vi "ConfigureDlg.vi"(8 "error in (no error)":errorcluster, 11 "MultiBandState in":refnum<class "MultiBandState.lvclass">) -> (0 "error out":errorcluster, 2 "Changed":bool, 3 "MultiBandState out":refnum<class "MultiBandState.lvclass">)   [LabVIEW 2014, in "Functions.lvlib" / "MultiBandState.lvclass"]
uses:
  MultiBandState.lvclass
  TypeDefs/clMultiBandConfig.ctl
  TypeDefs/MultiBandConfig.ctl
  MultiBandState.lvclass/MultiBandState.ctl
  FunctionBaseClass/FunctionBase.lvclass/FunctionBase.ctl
  FunctionBaseClass/Accessors/Read FunctionIniFilePath.vi
  Accessors/Write MultiBandConfig.vi
  Accessors/Read MultiBandConfig.vi
  <vilib>/Utility/config.llb/NI_LVConfig.lvlib
panel:
  in  "btnDone":bool
  in  "btnCancel":bool
  in  "MultiBandConfig":T1
  # "Band"
  # "Band"
  # "Band"
  # "Band"
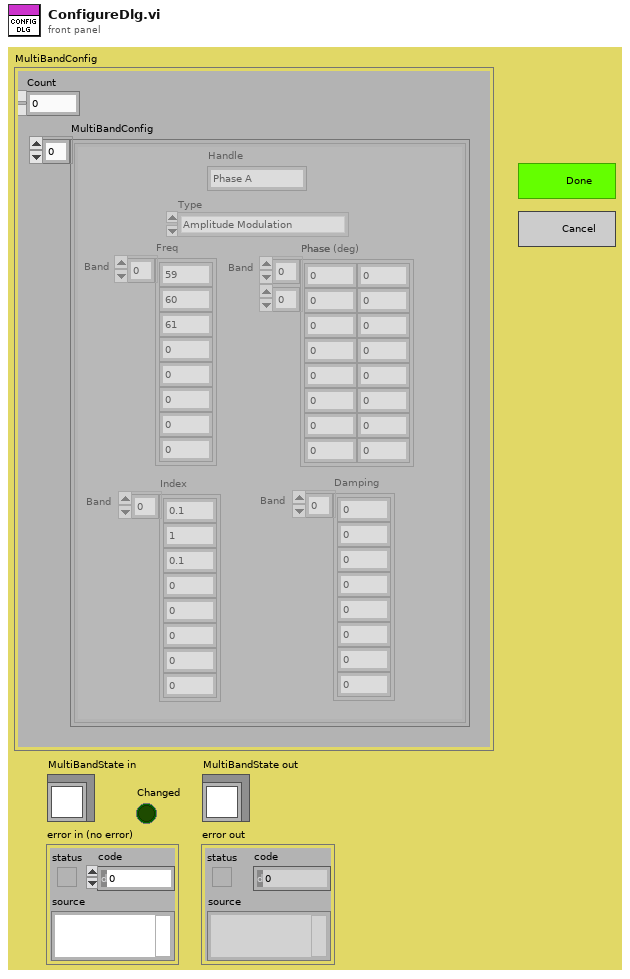
[diagram p1: front panel]
types:
  T1 = typedef "Functions.lvlib/MultiBandState.lvclass/clMultiBandConfig.ctl" = cluster{"Count":i32, "MultiBandConfig":T2[]}
  T2 = typedef "Functions.lvlib/MultiBandState.lvclass/MultiBandConfig.ctl" = cluster{"Handle":string, "Type":enum16{"Multiband", "Amplitude Modulation", "Phase Modulation", "Combined Modulation"}, "Freq":dbl[], "Index":dbl[], "Phase":dbl[][], "Damping":dbl[]}
  T3 = typedef "NI_LVConfig.lvlib/Config Data RefNum.ctl" = refnum<k1>
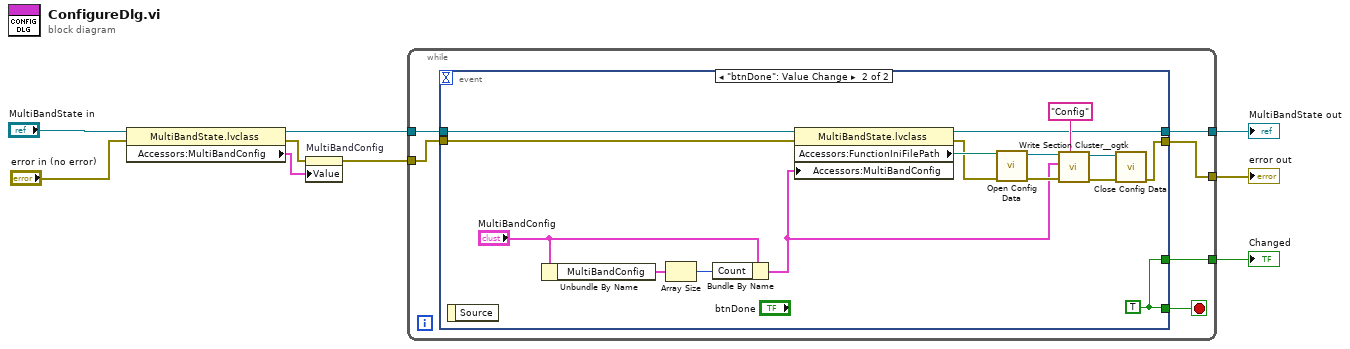
[diagram p0: block diagram]
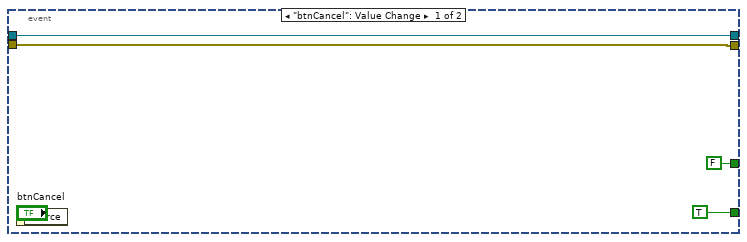
[diagram p2: hidden frame]
diagram:
  n1 = property class="MultiBandState.lvclass"(reference="MultiBandState in", error in="error in (no error)") -> (reference out=w7:refnum<class "MultiBandState.lvclass">, error out=w2:errorcluster, "Accessors:MultiBandConfig"=w3:T1)
  n2 = property on="MultiBandConfig" class="Clust (strict)"(error in=w2, "Value"=w3) -> (error out=w1:errorcluster)  [unwired: 1 in, 1 out]
  n3 = while {
    tunnel: w7 -> [w15]
    tunnel: [w14] -> w6
    tunnel: [w13] -> w5
    tunnel: [w11] -> w4
    tunnel: w1 -> [w10]
    stop <- w12 stop-if-true
    n4 = event shown="[1] \"btnDone\": Value Change" {
      selector: _ -> [_ _]
      dyn-events: _ -> [_ _]
      timeout: _ -> [_ _]
      tunnel: w15 -> [w19 w35]
      tunnel: [w19 w26] -> w14
      tunnel: w10 -> [w18 w24]
      tunnel: [w18 w25] -> w13
      tunnel: [TRUE w29] -> w12
      tunnel: [FALSE w29] -> w11
      event "btnCancel": Value Change {
        n5 = event-data() -> ()  [unwired: 1 in, 1 out]
      }
      event "btnDone": Value Change {
        w29 = TRUE
        n6 = event-data() -> ()  [unwired: 1 in, 1 out]
        n7 = Unbundle By Name("MultiBandConfig") -> ("MultiBandConfig"=w23:T2[])
        n8 = Array Size(array=w23) -> (size(s)=w22:i32)
        n9 = Bundle By Name(cluster="MultiBandConfig", "Count"=w22) -> (w20:T1)
        n10 = property class="MultiBandState.lvclass"(reference=w35, error in=w24, "Accessors:MultiBandConfig"=w20) -> (reference out=w26:refnum<class "MultiBandState.lvclass">, error out=w33:errorcluster, "Accessors:FunctionIniFilePath"=w34:path)
        n11 = call <vilib>:"Open Config Data.vi"("error in (no error)"=w33, "configuration file path"=w34) -> ("error out"=w28:errorcluster, "refnum"=w27:T3)  [unwired: 7 in, 1 out]
        n12 = call <userlib>:"Write Section Cluster__ogtk.vi"("section (optional)"="Config", "error in (no error)"=w28, "Section Formatted Cluster"=w20, "refnum"=w27) -> ("error out"=w31:errorcluster, "dup refnum"=w30:T3)  [unwired: 6 in]
        n13 = call <vilib>:"Close Config Data.vi"("error in (no error)"=w31, "refnum"=w30) -> ("error out"=w25:errorcluster)  [unwired: 8 in, 1 out]
      }
    }
  }
  "error out" <- w5
  "MultiBandState out" <- w6
  "Changed" <- w4
